vi "Launcher.vi"(8 "error in (no error)":errorcluster, 9 "Str Refnum":refnum<vi>, 10 "LaunchData":refnum<user-event>) -> (0 "error out":errorcluster, 3 "TopLevel out":refnum<class "TopLevel.lvclass">)   [LabVIEW 2022 SP3, in "TopLevel.lvclass"]
uses:
  TopLevel.lvclass
  DAQWFE/LV_Source/DataTypes/TD LaunchData--cluster.ctl
  DAQWFE/LV_Source/DataTypes/TD LaunchState--enum.ctl
  TopLevel_Process.vi
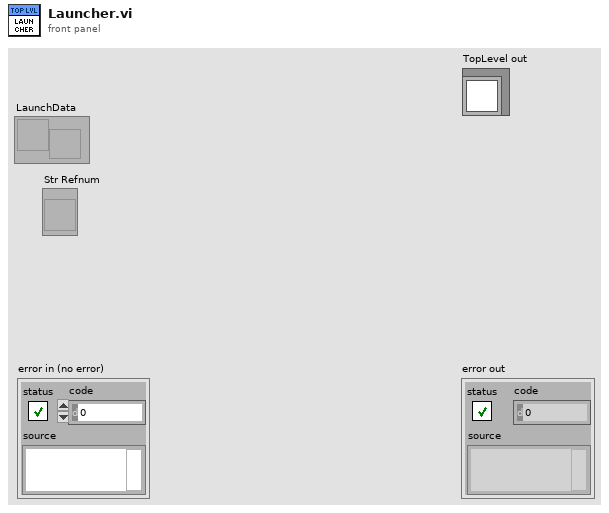
[diagram p1: front panel]
types:
  T1 = typedef "Rendezvous RefNum" = refnum<k1>
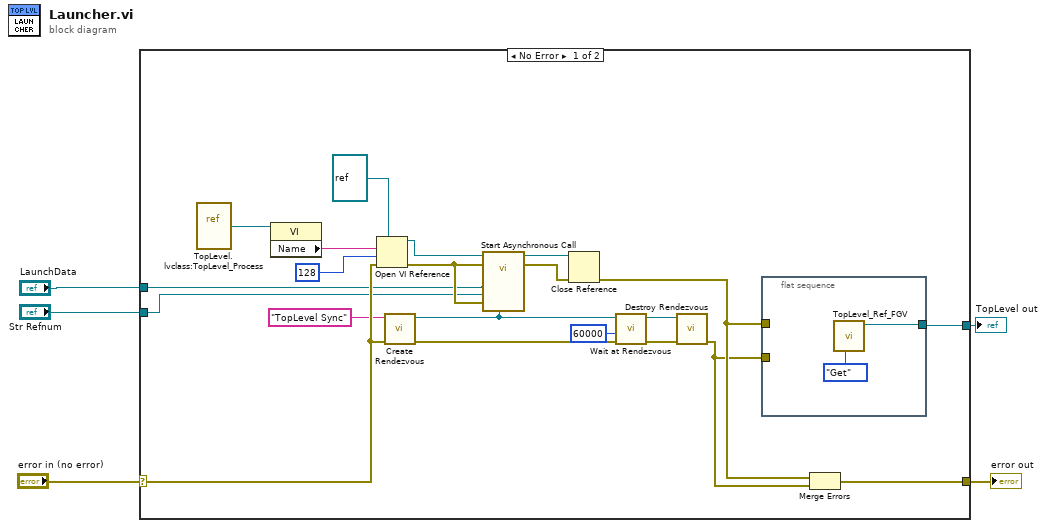
[diagram p0: block diagram]
diagram:
  n1 = case shown="No Error" "error in (no error)" {
    selector: "error in (no error)" -> [w22 w29]
    tunnel: [w11 w29] -> w4
    tunnel: [w10 _] -> w3
    tunnel: "LaunchData" -> [w7 _]
    tunnel: "Str Refnum" -> [w6 _]
    frame No Error {
      n2 = vi-ref "TopLevel.lvclass:TopLevel_Process.vi"() -> (w26:refnum<vi>)
      n3 = property class="VI"(reference=w26) -> ("Name"=w25:string)  [unwired: 1 in, 2 out]
      n4 = Open VI Reference(type specifier VI Refnum (for type only)=refnum<vi> refnum, vi path=w25, options=128, error in (no error)=w22) -> (vi reference=w21:refnum<vi>, error out=w20:errorcluster)  [unwired: 2 in]
      n5 = call <vilib>:"Create Rendezvous.vi"("error in (no error)"=w22, "name (unnamed)"="TopLevel Sync") -> ("error out"=w15:errorcluster, "rendezvous"=w16:T1)  [unwired: 3 in, 1 out]
      n6 = call-by-ref "Start Asynchronous Call"(reference=w21, error in=w20, "rendezvous ref"=w16, "error in"=w20, "Str Refnum"=w6, "LaunchData"=w7) -> (reference out=w19:refnum<vi>, error out=w18:errorcluster)  [unwired: 7 in, 1 out]
      n7 = Close Reference(reference=w19, error in (no error)=w18) -> (error out=w9:errorcluster)
      n8 = call <vilib>:"Wait at Rendezvous.vi"("error in (no error)"=w15, "ms timeout (-1)"=60000, "rendezvous"=w16) -> ("error out"=w12:errorcluster, "rendezvous out"=w13:T1)  [unwired: 2 in, 1 out]
      n9 = call <vilib>:"Destroy Rendezvous.vi"("error in (no error)"=w12, "rendezvous"=w13) -> ("error out"=w8:errorcluster)  [unwired: 4 in, 1 out]
      n10 = flat-sequence {
        tunnel: [w27] -> w10
        tunnel: w9 -> [_]
        tunnel: w8 -> [_]
        frame #0 {
          n11 = call "TopLevel_Ref_FGV.vi"("Action"=enum16{"Get", "Set", "Init"}."Get") -> ("TopLevel Out"=w27:refnum<class "TopLevel.lvclass">)  [unwired: 10 in]
        }
      }
      n12 = Merge Errors(w9, w8) -> (w11:errorcluster)
    }
    frame Error {
    }
  }
  "error out" <- w4
  "TopLevel out" <- w3
